vi "test_daqmx thermocouples pxi.vi"() -> ()   [LabVIEW 2023]
uses:
  Thermometer/Thermometer DAQmx Base CFG/Thermometer DAQmx Base CFG.lvclass
  Virtual Instrument Base/Virt Instr Base.lvclass
  <vilib>/Waveform/WDTOps.llb/WDT Number of Waveform Samples DBL.vi
  Measure and Stimulus Subsystems/Measure and Stimulus Subsystems.lvclass
panel:
  out "Lampentemp Chart":waveform(dbl)(graph)
  out "Tischtemp Chart":waveform(dbl)(graph)
  out "total samples fetched":i32
  out "#samples fetched":i32[](array[numeric])
  out "Iteration":i32
  in  "Stop":bool
  out "Error Out":errorcluster
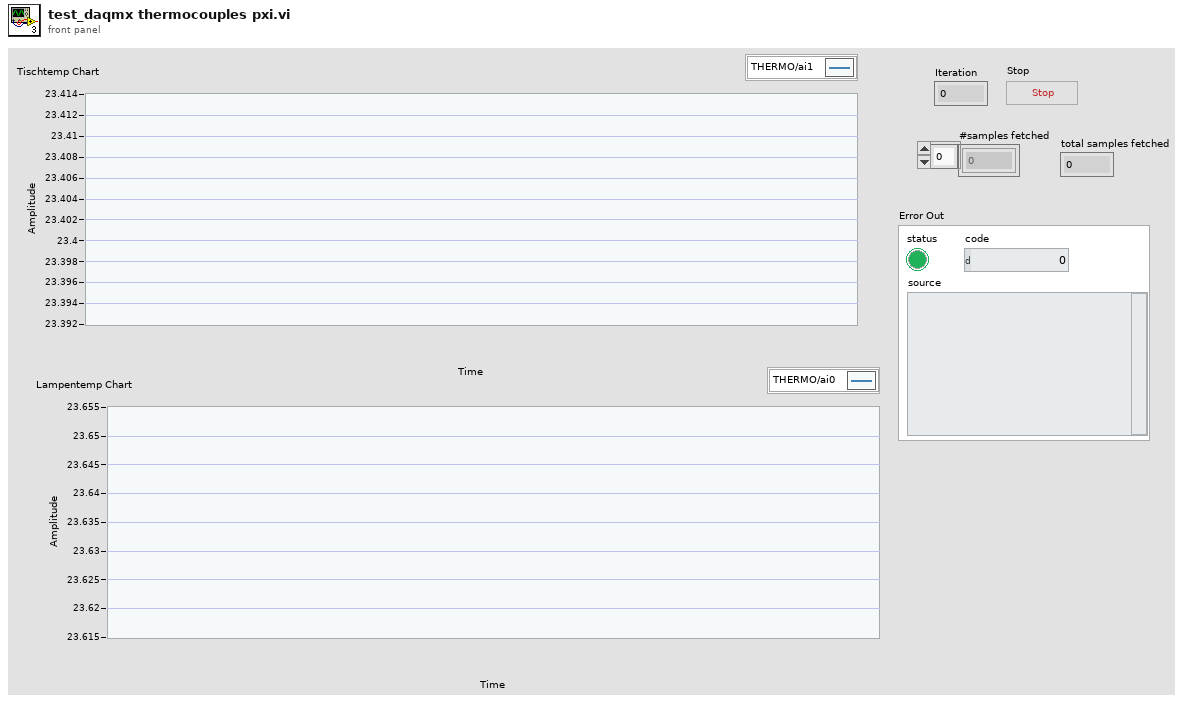
[diagram p1: front panel]
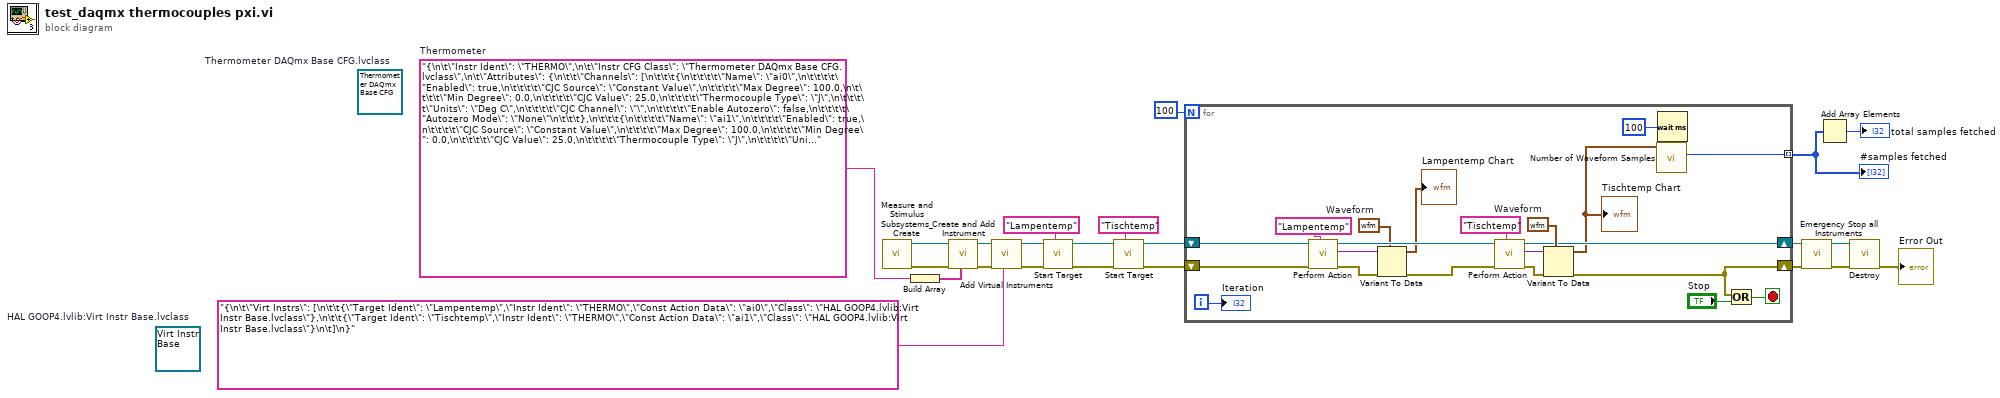
[diagram p0: block diagram]
diagram:
  (unwired) refnum<class "Virt Instr Base.lvclass"> refnum  # HAL GOOP4.lvlib:Virt Instr Base.lvclass
  (unwired) refnum<class "Thermometer DAQmx Base CFG.lvclass"> refnum  # Thermometer DAQmx Base CFG.lvclass
  w12 = "{\n\t\"Instr Ident\": \"THERMO\",\n\t\"Instr CFG Class\": \"Thermometer DAQmx Base CFG.lvclass\",\n\t\"Attributes\": {\n\t\t\"Channels\": [\n\t\t\t{\n\t\t\t\t\"Name\": \"ai0\",\n\t\t\t\t\"Enabled\": true,\n\t\t\t\t\"CJC Source\": \"Constant Value\",\n\t\t\t\t\"Max Degree\": 100.0,\n\t\t\t\t\"Min Degree\": 0.0,\n\t\t\t\t\"CJC Value\": 25.0,\n\t\t\t\t\"Thermocouple Type\": \"J\",\n\t\t\t\t\"Units\": \"Deg C\",\n\t\t\t\t\"CJC Channel\": \"\",\n\t\t\t\t\"Enable Autozero\": false,\n\t\t\t\t\"Autozero Mode\": \"None\"\n\t\t\t},\n\t\t\t{\n\t\t\t\t\"Name\": \"ai1\",\n\t\t\t\t\"Enabled\": true,\n\t\t\t\t\"CJC Source\": \"Constant Value\",\n\t\t\t\t\"Max Degree\": 100.0,\n\t\t\t\t\"Min Degree\": 0.0,\n\t\t\t\t\"CJC Value\": 25.0,\n\t\t\t\t\"Thermocouple Type\": \"J\",\n\t\t\t\t\"Units\": \"Deg C\",\n\t\t\t\t\"CJC Channel\": \"\",\n\t\t\t\t\"Enable Autozero\": false,\n\t\t\t\t\"Autozero Mode\": \"None\"\n\t\t\t},\n\t\t\t{\n\t\t\t\t\"Name\": \"ai2\",\n\t\t\t\t\"Enabled\": false,\n\t\t\t\t\"CJC Source\": \"Constant Value\",\n\t\t\t\t\"Max Degree\": 100.0,\n\t\t\t\t\"Min Degree\": 0.0,\n\t\t\t\t\"CJC Value\": 25.0,\n\t\t\t\t\"Thermocouple Type\": \"J\",\n\t\t\t\t\"Units\": \"Deg C\",\n\t\t\t\t\"CJC Channel\": \"\",\n\t\t\t\t\"Enable Autozero\": false,\n\t\t\t\t\"Autozero Mode\": \"None\"\n\t\t\t},\n\t\t\t{\n\t\t\t\t\"Name\": \"ai3\",\n\t\t\t\t\"Enabled\": false,\n\t\t\t\t\"CJC Source\": \"Constant Value\",\n\t\t\t\t\"Max Degree\": 100.0,\n\t\t\t\t\"Min Degree\": 0.0,\n\t\t\t\t\"CJC Value\": 25.0,\n\t\t\t\t\"Thermocouple Type\": \"J\",\n\t\t\t\t\"Units\": \"Deg C\",\n\t\t\t\t\"CJC Channel\": \"\",\n\t\t\t\t\"Enable Autozero\": false,\n\t\t\t\t\"Autozero Mode\": \"None\"\n\t\t\t},\n\t\t\t{\n\t\t\t\t\"Name\": \"ai4\",\n\t\t\t\t\"Enabled\": false,\n\t\t\t\t\"CJC Source\": \"Constant Value\",\n\t\t\t\t\"Max Degree\": 100.0,\n\t\t\t\t\"Min Degree\": 0.0,\n\t\t\t\t\"CJC Value\": 25.0,\n\t\t\t\t\"Thermocouple Type\": \"J\",\n\t\t\t\t\"Units\": \"Deg C\",\n\t\t\t\t\"CJC Channel\": \"\",\n\t\t\t\t\"Enable Autozero\": false,\n\t\t\t\t\"Autozero Mode\": \"None\"\n\t\t\t},\n\t\t\t{\n\t\t\t\t\"Name\": \"ai5\",\n\t\t\t\t\"Enabled\": false,\n\t\t\t\t\"CJC Source\": \"Constant Value\",\n\t\t\t\t\"Max Degree\": 100.0,\n\t\t\t\t\"Min Degree\": 0.0,\n\t\t\t\t\"CJC Value\": 25.0,\n\t\t\t\t\"Thermocouple Type\": \"J\",\n\t\t\t\t\"Units\": \"Deg C\",\n\t\t\t\t\"CJC Channel\": \"\",\n\t\t\t\t\"Enable Autozero\": false,\n\t\t\t\t\"Autozero Mode\": \"None\"\n\t\t\t},\n\t\t\t{\n\t\t\t\t\"Name\": \"ai6\",\n\t\t\t\t\"Enabled\": false,\n\t\t\t\t\"CJC Source\": \"Constant Value\",\n\t\t\t\t\"Max Degree\": 100.0,\n\t\t\t\t\"Min Degree\": 0.0,\n\t\t\t\t\"CJC Value\": 25.0,\n\t\t\t\t\"Thermocouple Type\": \"J\",\n\t\t\t\t\"Units\": \"Deg C\",\n\t\t\t\t\"CJC Channel\": \"\",\n\t\t\t\t\"Enable Autozero\": false,\n\t\t\t\t\"Autozero Mode\": \"None\"\n\t\t\t},\n\t\t\t{\n\t\t\t\t\"Name\": \"ai7\",\n\t\t\t\t\"Enabled\": false,\n\t\t\t\t\"CJC Source\": \"Constant Value\",\n\t\t\t\t\"Max Degree\": 100.0,\n\t\t\t\t\"Min Degree\": 0.0,\n\t\t\t\t\"CJC Value\": 25.0,\n\t\t\t\t\"Thermocouple Type\": \"J\",\n\t\t\t\t\"Units\": \"Deg C\",\n\t\t\t\t\"CJC Channel\": \"\",\n\t\t\t\t\"Enable Autozero\": false,\n\t\t\t\t\"Autozero Mode\": \"None\"\n\t\t\t}\n\t\t],\n\t\t\"Timing\": {\n\t\t\t\"Samples per Channel\": 1000,\n\t\t\t\"Sample Mode\": \"Continuous Samples\",\n\t\t\t\"Sample Rate\": 20.0,\n\t\t\t\"Sample Clock Source\": \"OnboardClock\",\n\t\t\t\"Active Edge\": \"Rising\"\n\t\t},\n\t\t\"Trigger\": {\n\t\t\t\"Trigger Type\": \"No Trigger\"\n\t\t},\n\t\t\"Acquisition\": {\n\t\t\t\"Relative To\": \"Current Read Position\",\n\t\t\t\"Overwrite\": \"Do Not Overwrite Unread Samples\",\n\t\t\t\"Samples per Fetch\": -1,\n\t\t\t\"Timeout\": 1.0\n\t\t}\n\t}\n}"  # Thermometer
  n1 = call "Measure and Stimulus Subsystems_Create.vi"() -> ("Error Out"=w22:errorcluster, "reference out"=w23:refnum<class "Measure and Stimulus Subsystems.lvclass">)  [unwired: 10 in]
  n2 = Build Array(w12) -> (w11:string[])
  n3 = call "Create and Add Instrument.vi"("Physical Intr Configs"=w11, "Error In"=w22, "reference in"=w23) -> ("Error Out"=w21:errorcluster, "reference out"=w3:refnum<class "Measure and Stimulus Subsystems.lvclass">)  [unwired: 7 in]
  n4 = call "Add Virtual Instruments.vi"("<JSON CFG>"="{\n\t\"Virt Instrs\": [\n\t\t{\"Target Ident\": \"Lampentemp\",\"Instr Ident\": \"THERMO\",\"Const Action Data\": \"ai0\",\"Class\": \"HAL GOOP4.lvlib:Virt Instr Base.lvclass\"},\n\t\t{\"Target Ident\": \"Tischtemp\",\"Instr Ident\": \"THERMO\",\"Const Action Data\": \"ai1\",\"Class\": \"HAL GOOP4.lvlib:Virt Instr Base.lvclass\"}\n\t]\n}", "Error In"=w21, "reference in"=w3) -> ("Error Out"=w5:errorcluster, "reference out"=w4:refnum<class "Measure and Stimulus Subsystems.lvclass">)  [unwired: 7 in]
  n5 = call "Start Target.vi"("Target Ident"="Lampentemp" ("Target Identifier"), "Error In"=w5, "reference in"=w4) -> ("Error Out"=w14:errorcluster, "reference out"=w8:refnum<class "Measure and Stimulus Subsystems.lvclass">)  [unwired: 7 in]
  n6 = call "Start Target.vi"("Target Ident"="Tischtemp", "Error In"=w14, "reference in"=w8) -> ("Error Out"=w9:errorcluster, "reference out"=w7:refnum<class "Measure and Stimulus Subsystems.lvclass">)  [unwired: 7 in]
  n7 = for {
    N: 100 -> [_]
    shift-right: [w33] -> w16
    shift-left: w9 -> [w42]
    shift-right: [w31] -> w19
    shift-left: w7 -> [w35]
    tunnel: [w24] -> w1 mode=indexing
    i -> [w36]
    stop <- w37 stop-if-true
    w26 = waveform(dbl) {"t0"=timestamp(0 s since 1904-01-01), "dt"=1.0, "Y"=[]}  # Waveform
    w32 = waveform(dbl) {"t0"=timestamp(0 s since 1904-01-01), "dt"=1.0, "Y"=[]}  # Waveform
    n8 = call "Perform Action.vi"("Target Ident"="Lampentemp" ("Target Identifier"), "Error In"=w42, "reference in"=w35) -> ("Error Out"=w43:errorcluster, "Output"=w41:variant, "reference out"=w34:refnum<class "Measure and Stimulus Subsystems.lvclass">)  [unwired: 6 in]
    n9 = Variant To Data(error in=w43, type=w26, Variant=w41) -> (data=→"Lampentemp Chart":waveform(dbl), error out=w38:errorcluster)
    n10 = call "Perform Action.vi"("Target Ident"="Tischtemp", "Error In"=w38, "reference in"=w34) -> ("Error Out"=w29:errorcluster, "Output"=w30:variant, "reference out"=w31:refnum<class "Measure and Stimulus Subsystems.lvclass">)  [unwired: 6 in]
    n11 = Variant To Data(error in=w29, type=w32, Variant=w30) -> (data=w27:waveform(dbl), error out=w33:errorcluster)
    "Tischtemp Chart" <- w27
    n12 = call-poly <vilib>:"Number of Waveform Samples.vi"("waveform in"=w27) -> ("number of samples"=w24:i32)  [unwired: 8 in, 2 out]
    n13 = Wait (ms)(milliseconds to wait=u32 100) -> ()  [unwired: 1 out]
    n14 = Or(x=w33, y="Stop") -> (x .or. y?=w37:bool)
    "Iteration" <- w36
  }
  "#samples fetched" <- w1
  n15 = call "Emergency Stop all Instruments.vi"("Error In"=w16, "reference in"=w19) -> ("Error Out"=w20:errorcluster, "reference out"=w18:refnum<class "Measure and Stimulus Subsystems.lvclass">)  [unwired: 8 in]
  n16 = Add Array Elements(numeric array=w1) -> (sum=→"total samples fetched":i32)
  n17 = call "Destroy.vi"("Error In"=w20, "reference in"=w18) -> ("Error Out"=→"Error Out":errorcluster)  [unwired: 8 in, 1 out]
